vi "Run Step.vi"(8 "error in (no error)":errorcluster, 10 "New Step":bool, 11 "Wait Step in":refnum<class "Wait Step Config.lvclass">) -> (0 "error out":errorcluster, 2 "Completed":bool, 3 "Wait Step out":refnum<class "Wait Step Config.lvclass">)   [LabVIEW 2015]
uses:
  Wait Step Config.lvclass
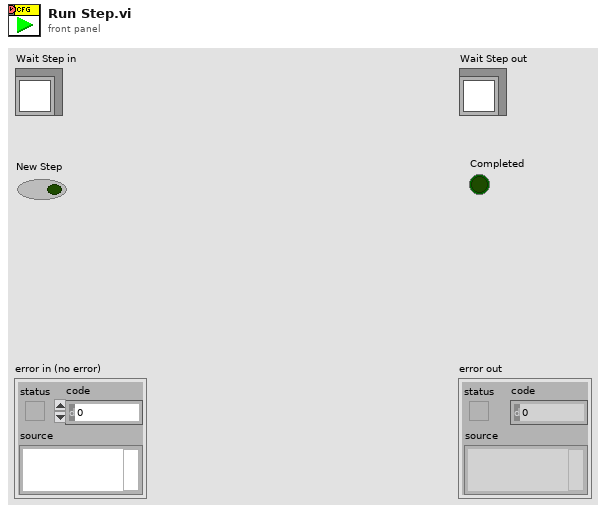
[diagram p1: front panel]
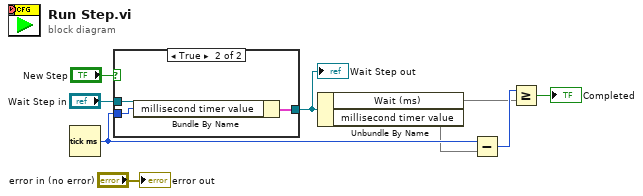
[diagram p0: block diagram]
diagram:
  n1 = Tick Count (ms)() -> (millisecond timer value=w5:u32)
  n2 = case shown="True" "New Step" {
    tunnel: w5 -> [_ w11]
    tunnel: "Wait Step in" -> [w10 w13]
    tunnel: [w10 w12] -> w6
    frame False {
    }
    frame True {
      n3 = Bundle By Name(cluster=w13, "millisecond timer value"=w11) -> (w12:cluster{})
    }
  }
  "Wait Step out" <- w6
  n4 = Unbundle By Name(w6) -> ("Wait (ms)"=w2, "millisecond timer value"=w4)
  n5 = Subtract(x=w5, y=w4) -> (x-y=w3:u32)
  n6 = Greater Or Equal?(x=w3, y=w2) -> (x >= y?=→"Completed":bool)
  "error out" <- "error in (no error)"
